vi "1K pot drain.vi"() -> ()   [LabVIEW 2021]
panel:
  in  "Still pressure threshold (mbar)":dbl format="%#_6e"
  in  "Fill voltage (V)":dbl
  in  "Drain voltage (V)":dbl
  # "Drains the 1K pot until the still pressure reaches\nthe threshold, then fills the 1K pot for 20 minutes\nbefore repeating the drain"
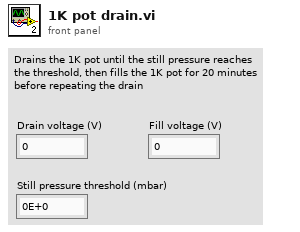
[diagram p1: front panel]
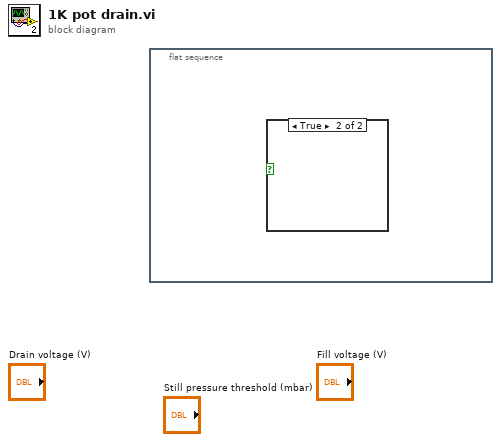
[diagram p0: block diagram]
diagram:
  n1 = flat-sequence {
    frame #0 {
      n2 = case shown="True" {
        selector: _ -> [_ _]
        frame False {
        }
        frame True {
        }
      }
    }
  }
